vi "Compile Incoming Frames.vi"(7 "Lookups in":variant, 8 "error in (no error)":errorcluster, 9 "Frame Settings Array":T3[](array[typedef]) {"Signals"."Byte Order" items=["Little Endian", "Big Endian"]; "Signals"."Data Type" items=["Signed", "Unsigned", "IEEE Float"]}, 10 "Refs":T1[](array[typedef]) {"Signal Refs" format="%.0x"}, 11 "Item Ref in":T2 format="%.0x") -> (0 "error out":errorcluster, 2 "Refs":T6[](array[typedef]) format="%.0x", 3 "Item Ref out":T2=18446744073709551615 format="%.0x", 5 "Lookups":variant)   [LabVIEW 2015, in "Diagnostics Addon System Explorer.lvlib"]
uses:
  Diagnostics Addon System Explorer.lvlib
  <vilib>/NI Veristand/Custom Device API/Custom Device Item Ref.ctl
  <vilib>/NI Veristand/Custom Device API/Data Reference.ctl
  Shared/Types/Common Frame Parameters.ctl
  Shared/Types/MessageType Selector.ctl
  Shared/Types/Signal Parameters.ctl
  Types/Frame Signal VS References.ctl
  <vilib>/NI Veristand/Custom Device API/Data Access Type.ctl
  Shared/Types/Datatable Lookup Positions.ctl
  Shared/Diagnostics Addon Shared.lvlib
  <vilib>/NI Veristand/Custom Device API/Custom Device API.lvlib
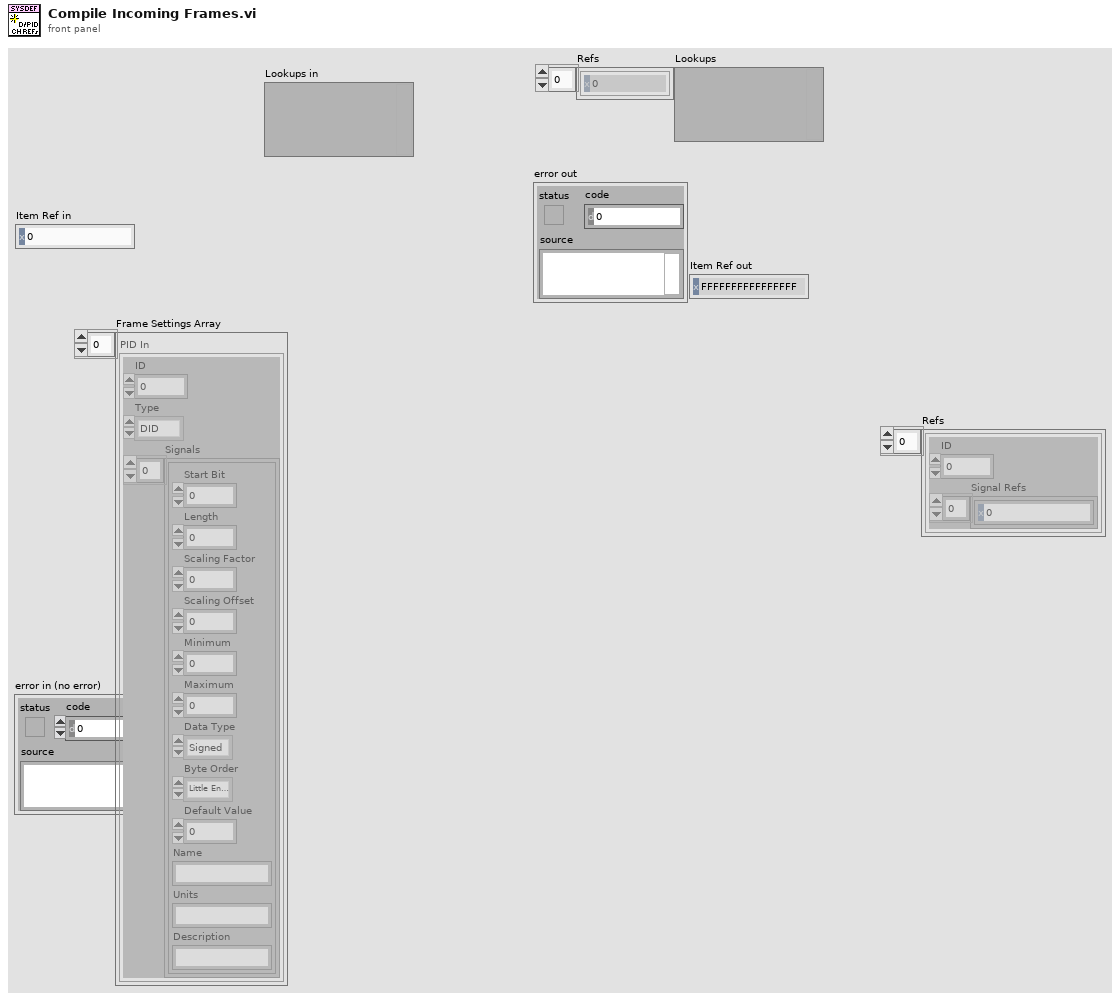
[diagram p1: front panel]
types:
  T1 = typedef "Diagnostics Addon System Explorer.lvlib/Frame Signal VS References.ctl" = cluster{"ID":u32, "Signal Refs":T2[]}
  T2 = typedef "Custom Device API.lvlib/Custom Device Item Ref.ctl" = u64
  T3 = typedef "Diagnostics Addon Shared.lvlib/Common Frame Parameters.ctl" = cluster{"ID":u32, "Type":T4, "Signals":T5[]}
  T4 = typedef "Diagnostics Addon Shared.lvlib/MessageType Selector.ctl" = enum16{"DID", "CDID", "PID", "CPID", "Read Memory", "Write Memory", "DTC Control", "IO Cmd", "IO Resp", "Routine Start Cmd", "Routine Start Resp", "Routine Request Cmd", "Routine Request Resp", "Routine Stop Cmd", "Routine Stop Resp"}
  T5 = typedef "Diagnostics Addon Shared.lvlib/Signal Parameters.ctl" = cluster{"Start Bit":u8, "Length":u8, "Scaling Factor":dbl, "Scaling Offset":dbl, "Minimum":dbl, "Maximum":dbl, "Data Type":u32, "Byte Order":u32, "Default Value":dbl, "Name":string, "Units":string, "Description":string}
  T6 = typedef "Custom Device API.lvlib/Data Reference.ctl" = i32
  T7 = typedef "Custom Device API.lvlib/Data Access Type.ctl" = enum16{"Read", "Write"}
  T8 = typedef "Diagnostics Addon Shared.lvlib/Datatable Lookup Positions.ctl" = cluster{"Offset":i32, "Length":i32, "ByteLength":u16}
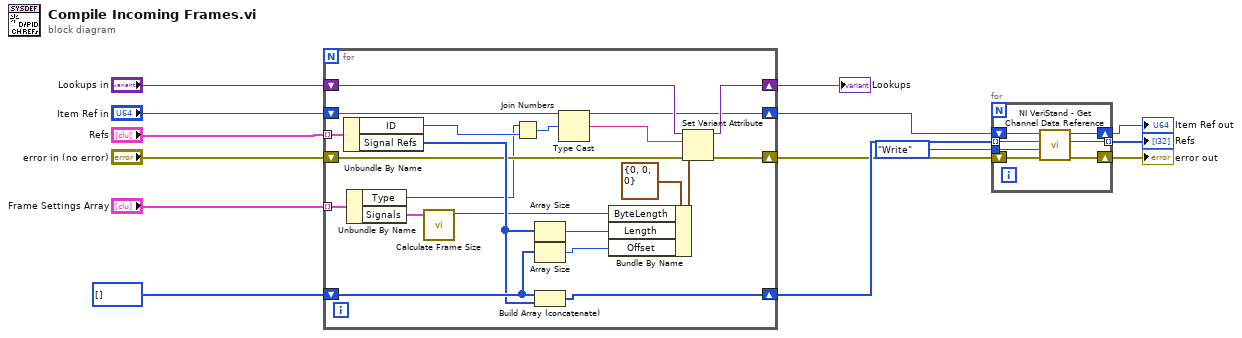
[diagram p0: block diagram]
diagram:
  n1 = for {
    tunnel: "Refs" -> [w24] mode=indexing
    shift-right: [w33] -> w9
    shift-left: T2[] [] ("Signal Refs") -> [w34]
    shift-right: [w25] -> w4
    shift-left: "Lookups in" -> [w29]
    shift-right: [w27] -> w8
    shift-left: "error in (no error)" -> [w22]
    shift-right: [w21] -> w10
    shift-left: "Item Ref in" -> [w21]
    tunnel: "Frame Settings Array" -> [w20] mode=indexing
    n2 = Unbundle By Name(w24) -> ("ID"=w17:u32, "Signal Refs"=w23:T2[])
    n3 = Unbundle By Name(w20) -> ("Type"=w15:T4, "Signals"=w19:T5[])
    n4 = call "Calculate Frame Size.vi"("Parameters"=w19) -> ("Bytes"=w18:u16)  [unwired: 10 in]
    n5 = Join Numbers(hi=w15, lo=w17) -> ((hi.lo)=w16:u64)
    n6 = Array Size(array=w23) -> (size(s)=w32:i32)
    n7 = Array Size(array=w34) -> (size(s)=w28:i32)
    n8 = Build Array (concatenate)(w34, w23) -> (w33:T2[])
    n9 = Type Cast(x=w16) -> (*(type *) &x=w26:string)  [unwired: 1 in]
    n10 = Bundle By Name(cluster=T8 {"Offset"=0, "Length"=0, "ByteLength"=0}, "ByteLength"=w18, "Length"=w32, "Offset"=w28) -> (w30:T8)
    n11 = Set Variant Attribute(Variant=w29, name=w26, value=w30, error in=w22) -> (Variant out=w25:variant, error out=w27:errorcluster)  [unwired: 1 out]
  }
  "Lookups" <- w4
  n12 = for {
    tunnel: w9 -> [w37] mode=indexing
    tunnel: Data_Access_Type."Write" ("Access") -> [w36]
    shift-right: [w39] -> w7
    shift-left: w8 -> [w40]
    shift-right: [w41] -> w6
    shift-left: w10 -> [w38]
    tunnel: [w35] -> w5 mode=indexing
    n13 = call <vilib>:"NI VeriStand - Get Channel Data Reference.vi"("error in (no error)"=w40, "Access"=w36, "Channel Ref in"=w37, "Device Ref in"=w38) -> ("error out"=w39:errorcluster, "Channel Data Reference"=w35:T6, "Device Ref out"=w41:T2)  [unwired: 5 in]
  }
  "error out" <- w7
  "Item Ref out" <- w6
  "Refs" <- w5
